vi "AudioTest.SoundCheck Data Log Analysis.vi"(11 "SoundCheck Data File":path) -> (0 "Error":errorcluster, 3 "Record Cnt":i32)   [LabVIEW 2018]
uses:
  TypeDefs/AudioTest.Analysis Data Record.ctl
  Common/Utils/Errors/Error.Error Code List.ctl
panel:
  in  "Exit":bool
  in  "Prev":bool
  in  "Next":bool
  out "Data":dbl[][](array[numeric])
  out "X Units":string
  out "Y Units":string
  out "XY Graph":cluster{"X":dbl[], "Y":dbl[]}(graph)
  in  "Load File":bool
  in  "Select Plot":u16(ring) items=["Spectrum [Reference Mic] (NOISE_FLOOR)", "Fundamental [Reference Mic] (LEFTr)", "Fundamental [DUT Mic] (RIGHTr)", "Fundamental [Reference Mic] (RON_LMICr)", "Fundamental [DUT Mic] (LON_RMICr)", "THD Normalized [Reference Mic] (LEFTr)", "Rub & Buzz Normalized [Reference Mic] (LEFTr)", "Rub & Buzz [Reference Mic] (LEFTr)", "Perceptual Rub & Buzz [Reference Mic] (LEFTr)", "THD Normalized [DUT Mic] (RIGHTr)", "Rub & Buzz Normalized [DUT Mic] (RIGHTr)", "Rub & Buzz [DUT Mic] (RIGHTr)", "Perceptual Rub & Buzz [DUT Mic] (RIGHTr)", "Fundamental [UTAH Left Mic] (L_UTAH_MICr)", "THD Normalized [UTAH Left Mic] (L_UTAH_MICr)", "THD [UTAH Left Mic] (L_UTAH_MICr)", "Rub & Buzz [UTAH Left Mic] (L_UTAH_MICr)", "Perceptual Rub & Buzz [UTAH Left Mic] (L_UTAH_MICr)", "LEFT_3rd", "RIGHT_3rd", "L_UTAH_MIC_3rd", "AVG_L_UTAH_MIC_3rd", "AVG_LEFT", "AVG_RIGHT", "AVG_RON_LMIC", "AVG_LON_RMIC", "LR_LEVEL_MATCH", "LEFT_CHAN_ON_OFF", "R_CHAN_ON_OFF", "LR_LEVEL_MATCH_MICS", "NOISE FLOOR Upper Limit [Reference Mic]", "LEFT_SENSITIVITY Upper Limit", "LEFT_SENSITIVITY Lower Limit", "RIGHT_SENSITIVITY Upper Limit", "RIGHT_SENSITIVITY Lower Limit", "CHANNEL_BALANCE Upper Limit", "CHANNEL_BALANCE Lower Limit", "LEFT_ASSIGNMENT Lower Limit", "RIGHT_ASSIGNMENT Lower Limit", "LEFT_MIC_SENSITIVITY Upper Limit", "LEFT_MIC_SENSITIVITY Lower Limit", "LEFT_POLARITY Lower Limit [Reference Mic]", "RIGHT_POLARITY Lower Limit [DUT Mic]", "LEFT_MIC_POLARITY Lower Limit [UTAH Left Mic]", "LEFT_3rd_SHAPE Upper Limit", "LEFT_3rd_SHAPE Lower Limit", "RIGHT_3rd_SHAPE Upper Limit", "RIGHT_3rd_SHAPE Lower Limit", "Norm_THD_LEFT Upper Limit [Reference Mic]", "Norm_THD_RIGHT Upper Limit [DUT Mic]", "PerceptualRUBBUZZ_LEFT Upper Limit [Reference Mic]", "PerceptualRUBBUZZ_RIGHT Upper Limit [DUT Mic]", "NormRUBBUZZ_LEFT Upper Limit [Reference Mic]", "NormRUBBUZZ_RIGHT Upper Limit [DUT Mic]", "LEFT_MIC_3rd_SHAPE Upper Limit", "LEFT_MIC_3rd_SHAPE Lower Limit", "Norm_THD_LEFT_MIC Upper Limit [UTAH Left Mic]"]
  # "Sound Check Data Analysis"
  # "X                    Y"
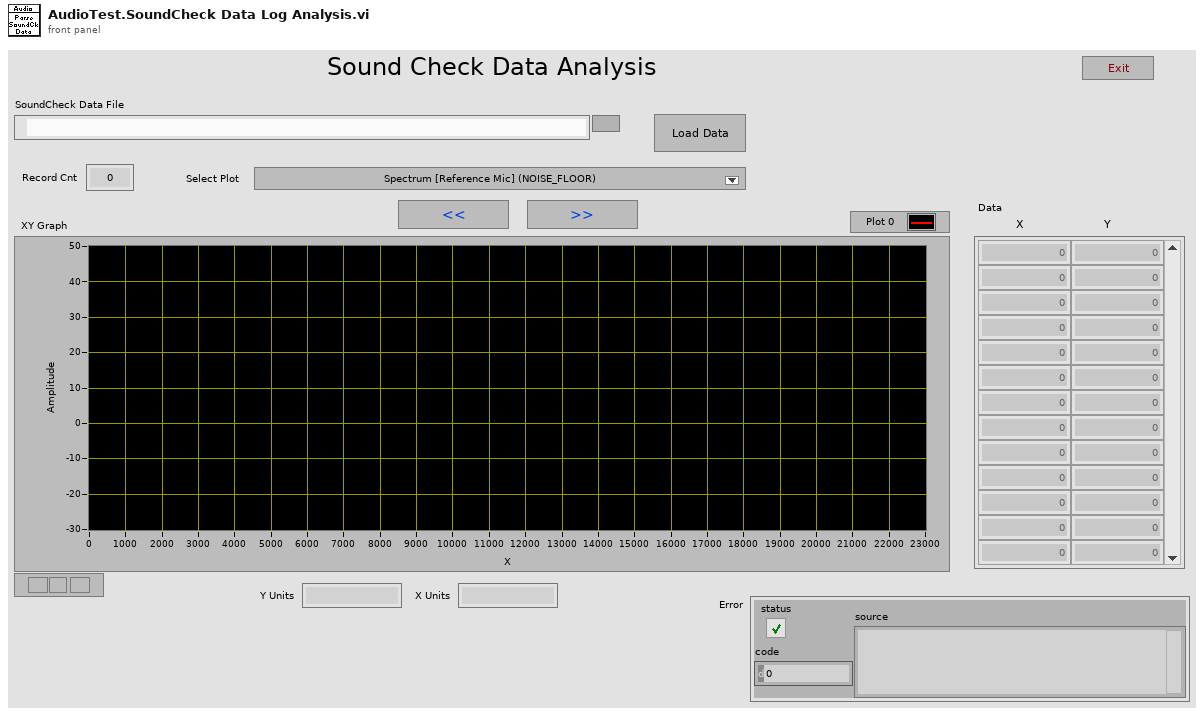
[diagram p1: front panel]
types:
  T1 = enum32{"invalid app kind", "Development System", "Run Time System", "Student Edition", "Embedded LabVIEW", "Evaluation", "Custom"}
  T2 = typedef "AudioTest.Analysis Data Record.ctl" = cluster{"Name":string, "X Units":string, "Y Units":string, "DataPlots":cluster{"X":dbl[], "Y":dbl[]}[], "LimitPlots":cluster{"X":dbl[], "Y":dbl[]}[], "DataPlotNames":string[], "LimitPlotNames":string[], "Fail":bool}
  T3 = typedef "Error.Error Code List.ctl" = i32
  T4 = typedef "Result.Attribute.ctl" = cluster{"Cnt":i32, "Step":string, "Category":string, "Name":string, "Value":string, "Status":T5, "Code":i32, "Desc":string, "Time":timestamp}
  T5 = typedef "Result.Measurement and Attribute Item Status.ctl" = i32
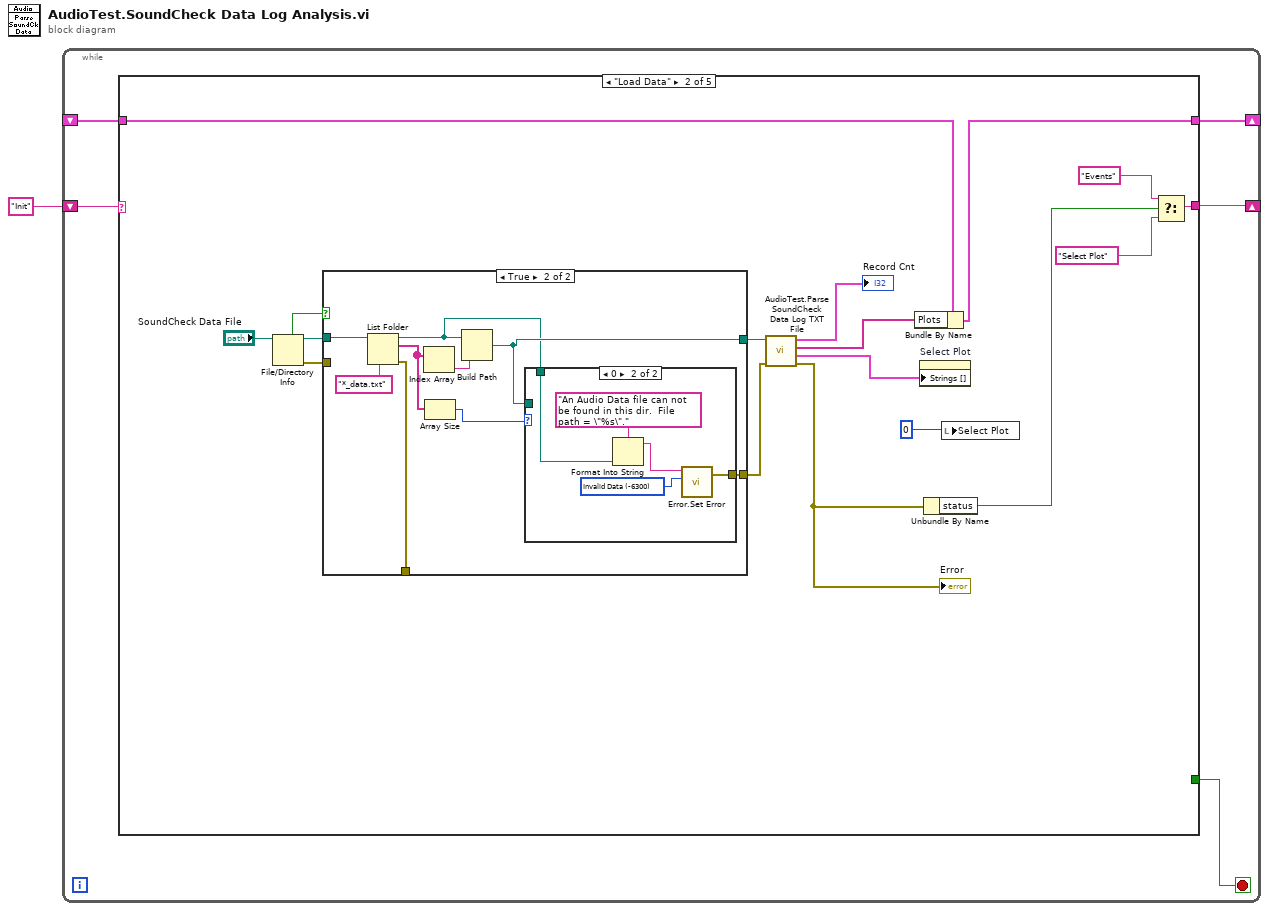
[diagram p0: block diagram]
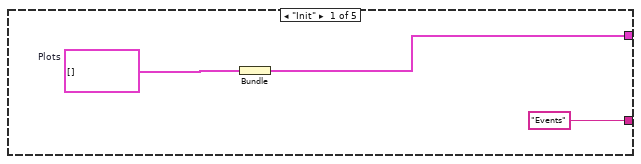
[diagram p2: hidden frame]
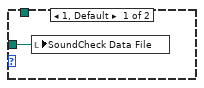
[diagram p4: hidden frame]
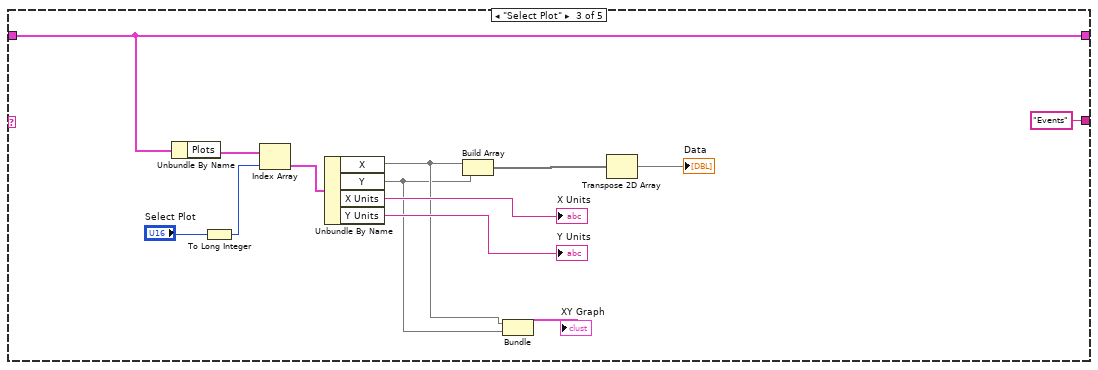
[diagram p5: hidden frame]
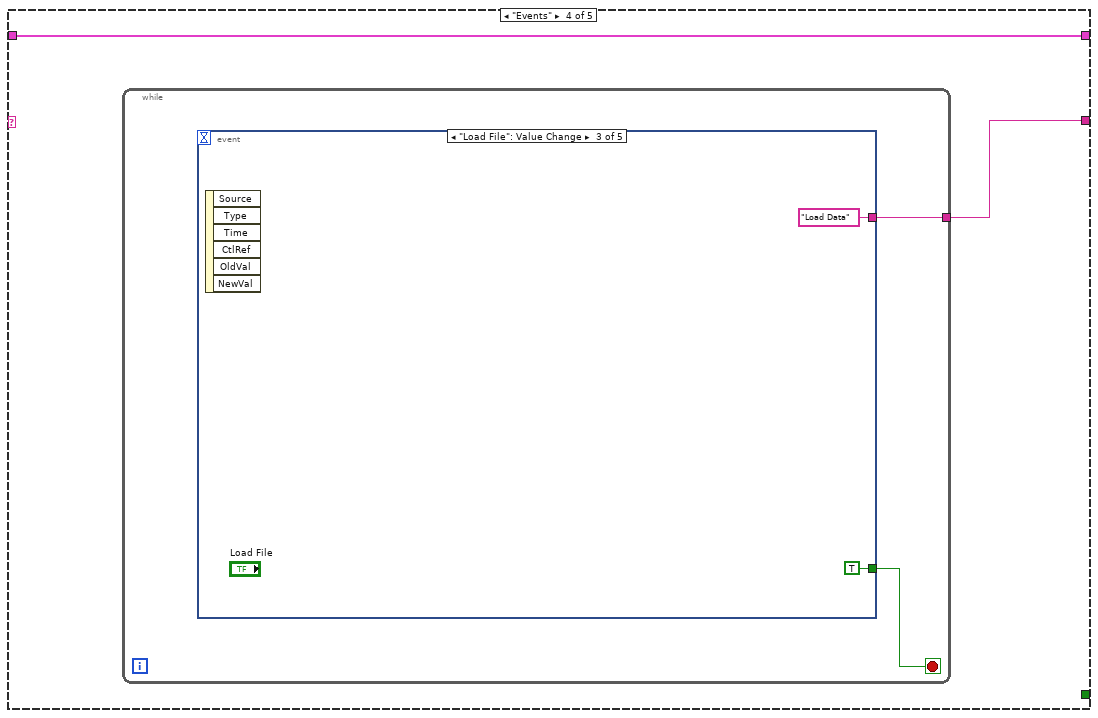
[diagram p6: hidden frame]
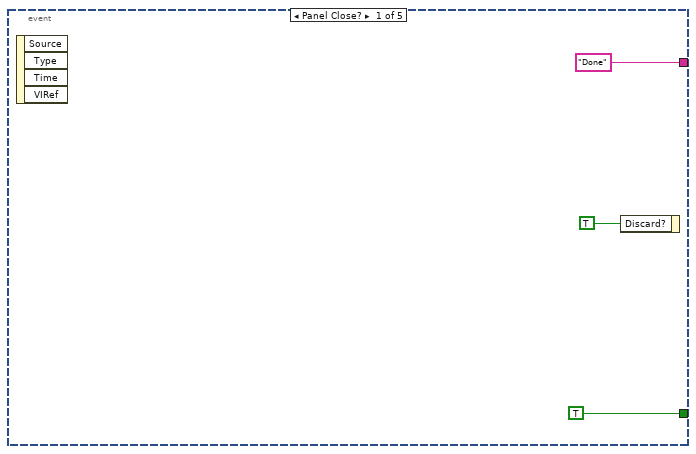
[diagram p7: hidden frame]
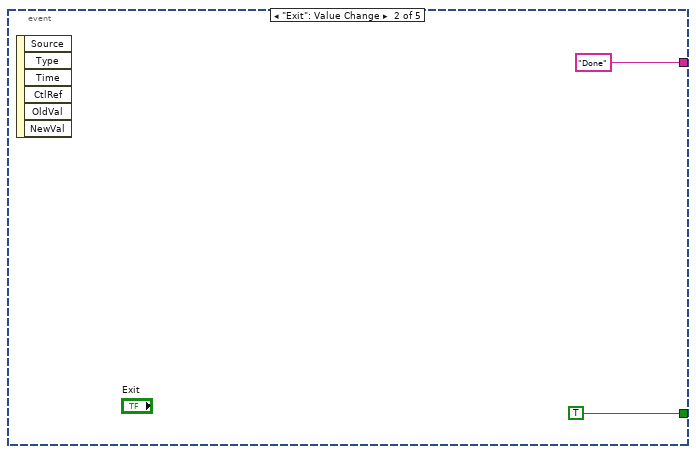
[diagram p8: hidden frame]
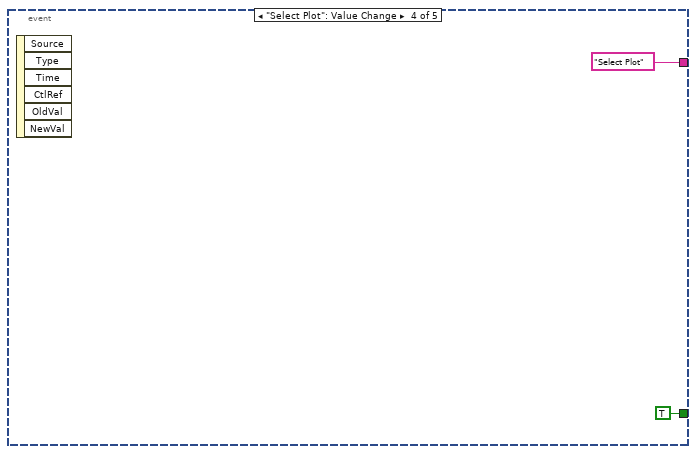
[diagram p9: hidden frame]
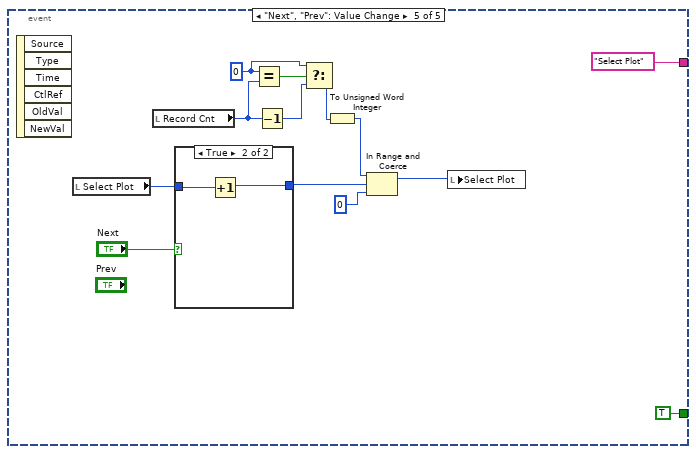
[diagram p10: hidden frame]
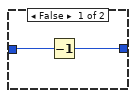
[diagram p11: hidden frame]
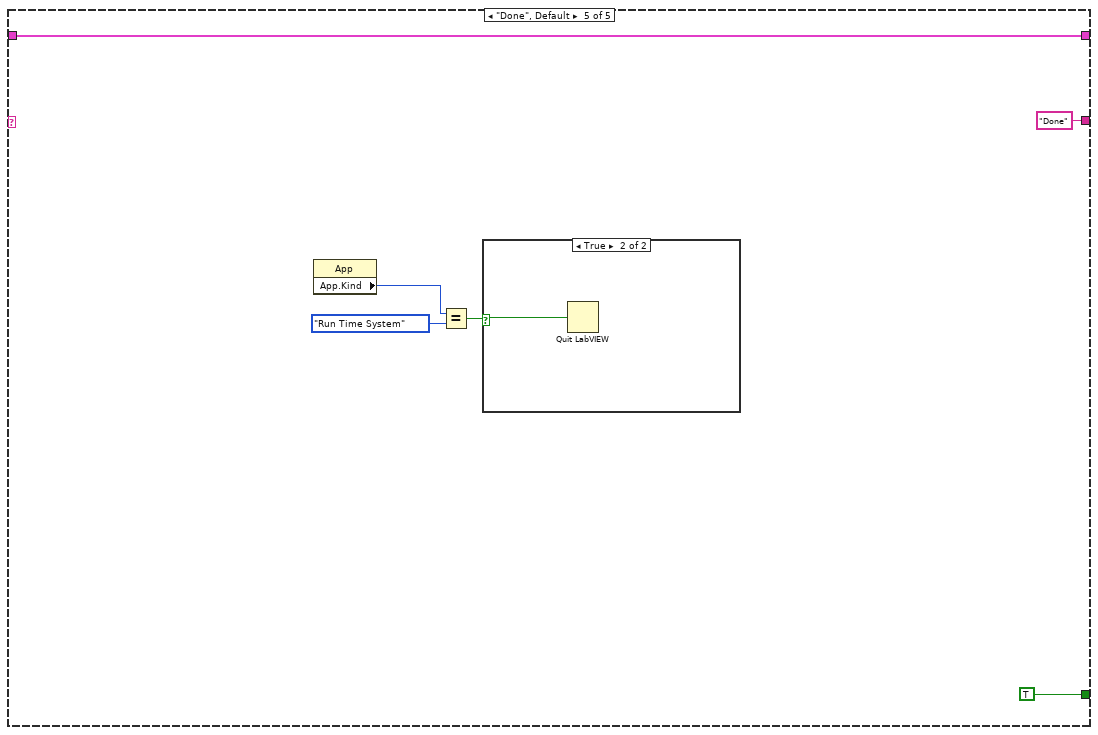
[diagram p12: hidden frame]
diagram:
  n1 = while {
    shift-right: [w6] -> _
    shift-left: _ -> [w3]
    shift-right: [w4] -> _
    shift-left: "Init" -> [w5]
    stop <- w2 stop-if-true
    n2 = case shown="\"Load Data\"" w5 {
      tunnel: [w7 w25 w54 w57 w90] -> w6
      tunnel: ["Events" w20 "Events" w56 "Done"] -> w4
      tunnel: w3 -> [_ w26 w54 w57 w90]
      tunnel: [_ _ _ _ TRUE] -> w2
      frame "Init" {
        w8 = T2[] []  # Plots
        n3 = Bundle("Plots"=w8) -> (w7:cluster{"Plots":T2[]})  [unwired: 1 in]
      }
      frame "Load Data" {
        n4 = File/Directory Info(path="SoundCheck Data File") -> (path out=w14:path, directory=w13:bool, error out=w11:errorcluster)  [unwired: 1 in, 4 out]
        n5 = case shown="True" w13 {
          tunnel: w14 -> [w27 w36]
          tunnel: [w27 w34] -> w12
          tunnel: w11 -> [_ _]
          tunnel: [_ w33] -> _
          tunnel: [_ w29] -> w10
          frame False {
          }
          frame True {
            n6 = List Folder(path=w36, pattern="*_data.txt") -> (path out=w28:path, filenames=w32:string[], error out=w33:errorcluster)  [unwired: 2 in, 1 out]
            n7 = Index Array(array=w32) -> (element=w30:string)  [unwired: 1 in]
            n8 = Array Size(array=w32) -> (size(s)=w31:i32)
            n9 = Build Path(base path=w28, name or relative path=w30) -> (appended path=w34:path)
            n10 = case shown="0" w31 {
              tunnel: w34 -> [w37 _]
              tunnel: [_ w39] -> w29
              tunnel: w28 -> [_ w38]
              frame 1, Default {
                n11 = local write "SoundCheck Data File"(w37) -> ()
              }
              frame 0 {
                w40 = T3 -6300 items=["No Error"=0, "Abort"=-2, "Misc"=-5000, "Fixture Error"=-5100, "File IO - General"=-5200, "FIle IO - Config Error"=-5201, "Instrument - General"=-5300, "Instrument - Serial Com"=-5301, "Instrument - Camera"=-5302, "Instrument - PS"=-5303, "Instrument - Oscilloscope"=-5304, "Instrument - Function Gen"=-5305, "Instrument - Load"=-5306, "Instrument - Meter"=-5307, "Instrument - Power Control"=-5308, "Instrument - Motion"=-5309, "Instrument - RF"=-5310, "System Exe"=-5400, "Image Processing"=-5500, "Communication"=-5600, "Script - Syntax Error"=-6000, "Script - Invalid Name or Param"=-6100, "Script - Timeout"=-6200, "Invalid Data"=-6300, "FW Update Error"=-6500] ("Std Code")
                n12 = Format Into String(format string="An Audio Data file can not be found in this dir.  File path = \"%s\"." ("Desc"), w38) -> (resulting string=w42:string)  [unwired: 2 in, 1 out]
                n13 = call "Error.Set Error.vi"("Code"=w40, "Desc"=w42) -> ("error out"=w39:errorcluster)  [unwired: 5 in]
              }
            }
          }
        }
        n14 = call "AudioTest.Parse SoundCheck Data Log TXT File.vi"("error in"=w10, "SoundCheck Data File"=w12) -> ("error out"=w17:errorcluster, "Attr Rslt"=w22:T4[], "Graph Names"=w24:string[], "Graphs"=→"Record Cnt":T2[])  [unwired: 5 in, 1 out]
        "Error" <- w17
        n15 = Bundle By Name(cluster=w26, "Plots"=w24) -> (w25:cluster{"Plots":T2[]})
        n16 = property on="Select Plot" class="Ring (strict)"("Strings []"=w22) -> ()  [unwired: 2 in, 2 out]
        n17 = Unbundle By Name(w17) -> ("status"=w16:bool)
        n18 = local write "Select Plot"(0) -> ()
        n19 = Select(t="Events", s=w16, f="Select Plot") -> (s? t:f=w20:string)
      }
      frame "Select Plot" {
        n20 = Unbundle By Name(w54) -> ("Plots"=w53:T2[])
        n21 = To Long Integer(number="Select Plot") -> (32bit integer=w50:i32)
        n22 = Index Array(array=w53, index=w50) -> (element=w52:T2)
        n23 = Unbundle By Name(w52) -> ("X"=w47, "Y"=w46, "X Units"=→"X Units":string, "Y Units"=→"Y Units":string)
        n24 = Build Array(w47, w46) -> (w44:void[])
        n25 = Bundle("X"=w47, "Y"=w46) -> (→"XY Graph":cluster{"X":void, "Y":void})  [unwired: 1 in]
        n26 = Transpose 2D Array(2D array=w44) -> (transposed array=→"Data":void[][])
      }
      frame "Events" {
        n27 = while {
          tunnel: [w58] -> w56
          stop <- w59 stop-if-true
          n28 = event shown="[2] \"Load File\": Value Change" {
            selector: _ -> [_ _ _ _ _]
            dyn-events: _ -> [_ _ _ _ _]
            timeout: _ -> [_ _ _ _ _]
            tunnel: [TRUE TRUE TRUE TRUE TRUE] -> w59
            tunnel: ["Done" "Done" "Load Data" "Select Plot" "Select Plot"] -> w58
            event Panel Close? {
              n29 = event-data() -> ()  [unwired: 1 in, 4 out]
              n30 = event-data("Discard?"=TRUE) -> ()  [unwired: 1 in, 1 out]
            }
            event "Exit": Value Change {
              n31 = event-data() -> ()  [unwired: 1 in, 6 out]
            }
            event "Load File": Value Change {
              n32 = event-data() -> ()  [unwired: 1 in, 6 out]
            }
            event "Select Plot": Value Change {
              n33 = event-data() -> ()  [unwired: 1 in, 6 out]
            }
            event "Next", "Prev": Value Change {
              w71 = 0 ("x")
              n34 = event-data() -> ()  [unwired: 1 in, 6 out]
              n35 = local read "Select Plot"() -> (w79:u16)
              n36 = local read "Record Cnt"() -> (w73:i32)
              n37 = case shown="True" "Next" {
                tunnel: w79 -> [w83 w85]
                tunnel: [w82 w84] -> w77
                frame False {
                  n38 = Decrement(x=w83) -> (x-1=w82:u16)
                }
                frame True {
                  n39 = Increment(x=w85) -> (x+1=w84:u16)
                }
              }
              n40 = Equal?(x=w71, y=w73) -> (x = y?=w72:bool)
              n41 = Decrement(x=w73) -> (x-1=w70:i32)
              n42 = Select(t=w71, s=w72, f=w70) -> (s? t:f=w69:i32)
              n43 = To Unsigned Word Integer(number=w69) -> (unsigned 16bit integer=w74:u16)
              n44 = In Range and Coerce(upper limit=w74, x=w77, lower limit=u16 0) -> (coerced(x)=w75:u16)  [unwired: 1 out]
              n45 = local write "Select Plot"(w75) -> ()
            }
          }
        }
      }
      frame "Done", Default {
        n46 = property class="App"() -> ("App.Kind"=w89:T1)  [unwired: 2 in, 2 out]
        n47 = Equal?(x=w89, y=T1."Run Time System") -> (x = y?=w87:bool)
        n48 = case shown="True" w87 {
          selector: w87 -> [_ w92]
          frame False {
          }
          frame True {
            n49 = Quit LabVIEW(quit? (T)=w92) -> ()
          }
        }
      }
    }
  }
